vi "setClaseEstadistica.vi"(8 "error in":errorcluster, 10 "dataToSet":T1, 11 "claseEstadistica in":refnum<class "claseEstadistica.lvclass">) -> (0 "error out":errorcluster, 3 "claseEstadistica out":refnum<class "claseEstadistica.lvclass">)   [LabVIEW 2014, in "claseEstadistica.lvclass"]
uses:
  claseEstadistica.lvclass
  claseEstadistica.lvclass/claseEstadistica.ctl
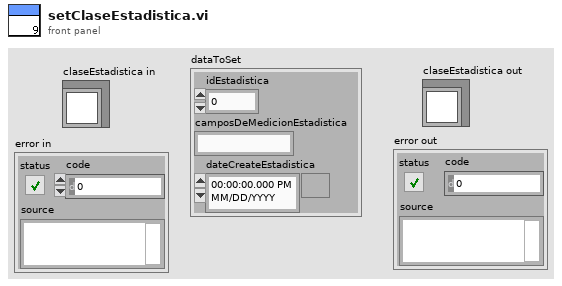
[diagram p1: front panel]
types:
  T1 = cluster{"idEstadistica":dbl, "camposDeMedicionEstadistica":string, "dateCreateEstadistica":timestamp}
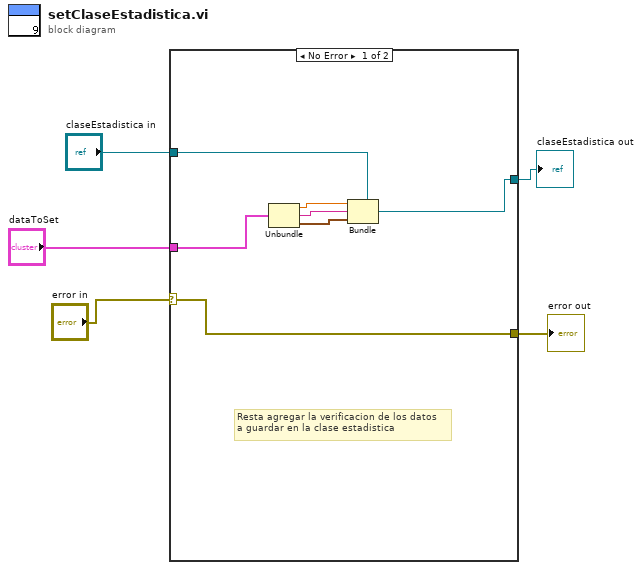
[diagram p0: block diagram]
diagram:
  n1 = case shown="No Error" "error in" {
    selector: "error in" -> [w12 w14]
    tunnel: [w12 w14] -> w4
    tunnel: [w10 w13] -> w3
    tunnel: "claseEstadistica in" -> [w11 w13]
    tunnel: "dataToSet" -> [w9 _]
    frame No Error {
      # "Resta agregar la verificacion de los datos\na guardar en la clase estadistica"
      n2 = Unbundle(w9) -> ("idEstadistica"=w8:dbl, "camposDeMedicionEstadistica"=w7:string, "dateCreateEstadistica"=w6:timestamp)
      n3 = Bundle(cluster=w11, w8, w7, w6) -> (w10:refnum<class "claseEstadistica.lvclass">)
    }
    frame Error {
    }
  }
  "claseEstadistica out" <- w3
  "error out" <- w4
